vi "Draw Waveforms.vi"(2 "Display State In":T1={"Show Axes"=FALSE, "Show Y=0"=FALSE, "Controls"={"Type"=enum."Sine", "Periods"=0.0, "Points"=0, "Offset"=0.0, "Amplitdue"=0.0, "Starting Phase"=0.0, "func"=""}, "Show Current Location"=FALSE, "Current Location"=0, "dt"=0.0, "t0"=timestamp(0 s since 1904-01-01), "Amplitude Format String"="%_3p"} caption="State" {"Controls"."Points" format="%_3p"}, 3 "Data In":T4) -> (0 "Display State Out":T1={"Show Axes"=FALSE, "Show Y=0"=FALSE, "Controls"={"Type"=enum."Sine", "Periods"=0.0, "Points"=0, "Offset"=0.0, "Amplitdue"=0.0, "Starting Phase"=0.0, "func"=""}, "Show Current Location"=FALSE, "Current Location"=0, "dt"=0.0, "t0"=timestamp(0 s since 1904-01-01), "Amplitude Format String"="%_3p"} caption="State" {"Controls"."Points" format="%_3p"}, 1 "Array":T4[](array[typedef]))   [LabVIEW 2018, in "Waveform Control.xctl"]
doc: "Creates an array of waveforms based on the input waveform + waveforms for the y=0 line and the current position marker if these are turned on in the XControl state cluster"
uses:
  Waveform Control.xctl
  Controls/Data.ctl
  Controls/Waveform State.ctl
  FP Controls.ctl
  Function Types.ctl
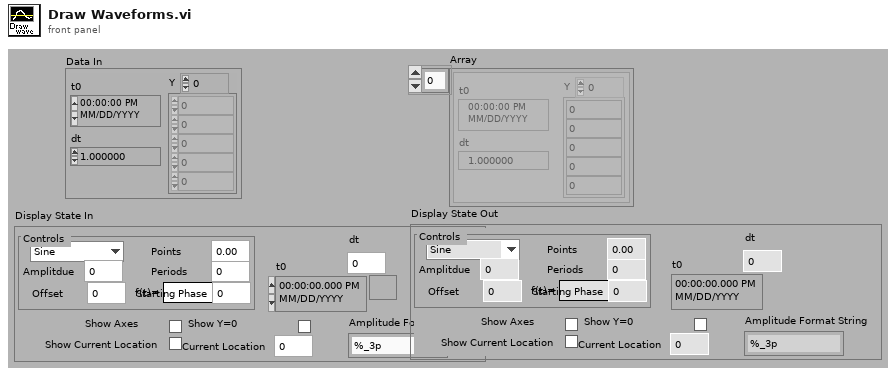
[diagram p1: front panel]
types:
  T1 = typedef "Waveform Control.xctl/Waveform State.ctl" = cluster{"Show Axes":bool, "Show Y=0":bool, "Controls":T2, "Show Current Location":bool, "Current Location":i32, "dt":dbl, "t0":timestamp, "Amplitude Format String":string}
  T2 = typedef "Waveform Control.xctl/FP Controls.ctl" = cluster{"Type":T3, "Periods":dbl, "Points":i32, "Offset":dbl, "Amplitdue":dbl, "Starting Phase":dbl, "func":string}
  T3 = typedef "Waveform Control.xctl/Function Types.ctl" = enum16{"Level", "Sine", "Triangle", "Ramp", "Saw Tooth", "Square", "Function"}
  T4 = typedef "Waveform Control.xctl/Data.ctl" = waveform(dbl)
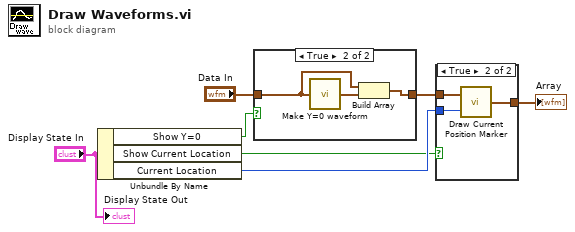
[diagram p0: block diagram]
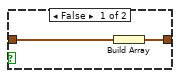
[diagram p3: hidden frame]
diagram:
  n1 = Unbundle By Name("Display State In") -> ("Show Y=0"=w2:bool, "Show Current Location"=w4:bool, "Current Location"=w5:i32)
  n2 = case shown="True" w2 {
    tunnel: [w8 w12] -> w6
    tunnel: "Data In" -> [w9 w11]
    frame False {
      n3 = Build Array(w9) -> (w8:T4[])
    }
    frame True {
      n4 = call "Make Y=0 waveform.vi"("signal out 2"=w11) -> ("signal out"=w10:waveform(dbl))
      n5 = Build Array(w11, w10) -> (w12:T4[])
    }
  }
  n6 = case shown="True" w4 {
    tunnel: w5 -> [_ w16]
    tunnel: w6 -> [w13 w15]
    tunnel: [w13 w14] -> w7
    frame False {
    }
    frame True {
      n7 = call "Draw Current Position Marker.vi"("Current Location"=w16, "Array 2"=w15) -> ("Array"=w14:T4[])
    }
  }
  "Array" <- w7
  "Display State Out" <- "Display State In"
